vi "FS Sketch Rectangle.vi"(8 "Sketch #":i32=1, 9 "rect":T2={"left"=0.0, "top"=0.0, "right"=3.0, "bottom"=4.0}, 10 "Sketch Plane":T1, 11 "Feature In":string="FeatureScript 1247;\nimport(path : \"onshape/std/geometry.fs\", version : \"1247.0\");\n\nannotation { \"Feature Type Name\" : \"LabVIEW Feature\" }\nexport const myFeature = defineFeature(function(context is Context, id is Id, definition is map)\n    precondition\n    {\n        // Define the parameters of the feature type\n    }\n    {\n        // Define the function's action\n    });") -> (3 "Feature Out":string="FeatureScript 1247;\nimport(path : \"onshape/std/geometry.fs\", version : \"1247.0\");\n\nannotation { \"Feature Type Name\" : \"LVFeat1\" }\nexport const myFeature = defineFeature(function(context is Context, id is Id, definition is map)\n    precondition\n    {\n        // Define the parameters of the feature type\n    }\n    {\n        // Define the function's action\n\nvar sketch1 = newSketch(context, id + \"sketch1\", {\n                \"sketchPlane\" : qCreatedBy(makeId(\"Top\"), EntityType.FACE)\n        });\n        // Create sketch entities here\n        skRectangle(sketch1, \"rectangle1\", {\n                \"firstCorner\" : vector(0, 0) * inch,\n                \"secondCorner\" : vector(3, 4) * inch\n        });\n        \n        skSolve(sketch1);\n    });")   [LabVIEW 2019]
uses:
  <userlib>/Onshape Feature Funcrions/_SubVI/Sketch Plane.ctl
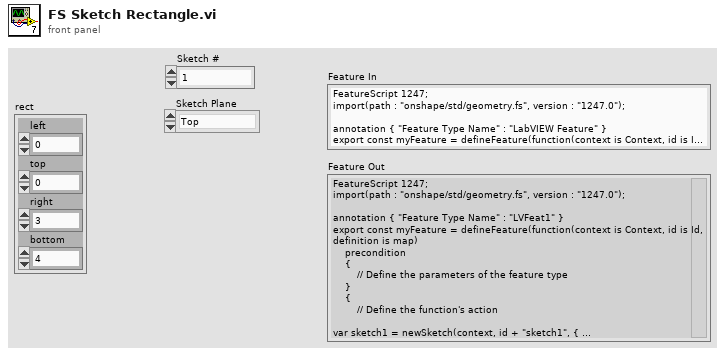
[diagram p1: front panel]
types:
  T1 = typedef "Sketch Plane.ctl" = enum16{"Top", "Front", "Right", "plane1", "plane2", "plane3"}
  T2 = cluster{"left":dbl, "top":dbl, "right":dbl, "bottom":dbl}
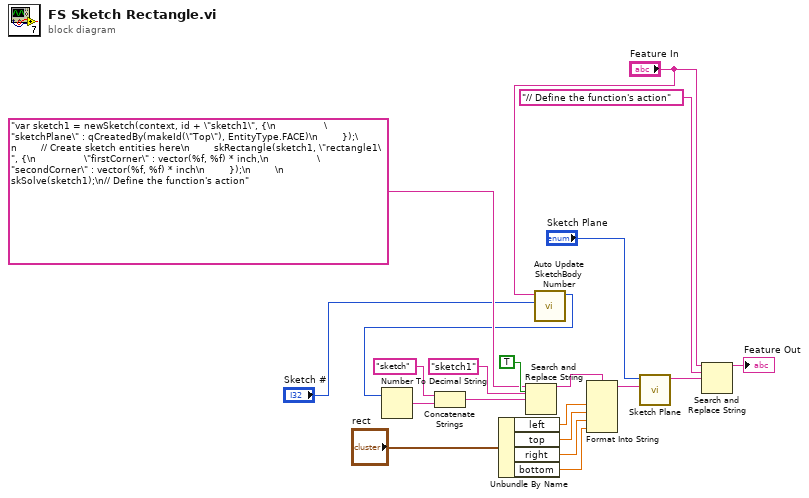
[diagram p0: block diagram]
diagram:
  n1 = Unbundle By Name("rect") -> ("left"=w11:dbl, "top"=w10:dbl, "right"=w9:dbl, "bottom"=w8:dbl)
  n2 = call "Auto Update SketchBody Number.vi"("Sketch # in"="Sketch #", "Feature In"="Feature In") -> ("Sketch # out"=w1:i32)  [unwired: 8 in, 1 out]
  n3 = Number To Decimal String(number=w1) -> (decimal integer string=w12:string)  [unwired: 1 in]
  n4 = Concatenate Strings("sketch" ("regular expression"), w12) -> (w14:string)
  n5 = Search and Replace String(replace all?=TRUE ("replace all? (F)"), input string="var sketch1 = newSketch(context, id + \"sketch1\", {\n                \"sketchPlane\" : qCreatedBy(makeId(\"Top\"), EntityType.FACE)\n        });\n        // Create sketch entities here\n        skRectangle(sketch1, \"rectangle1\", {\n                \"firstCorner\" : vector(%f, %f) * inch,\n                \"secondCorner\" : vector(%f, %f) * inch\n        });\n        \n        skSolve(sketch1);\n// Define the function's action", search string="sketch1" ("regular expression"), replace string=w14) -> (result string=w4:string)  [unwired: 4 in, 3 out]
  n6 = Format Into String(format string=w4, w11, w10, w9, w8) -> (resulting string=w7:string)  [unwired: 2 in, 1 out]
  n7 = call <userlib>:"Sketch Plane.vi"("result string in"=w7, "Sketch Plane"="Sketch Plane") -> ("result string out"=w6:string)  [unwired: 9 in]
  n8 = Search and Replace String(input string="Feature In", search string="// Define the function's action", replace string=w6) -> (result string=→"Feature Out":string)  [unwired: 5 in, 3 out]
